vi "lab2_4.vi"() -> ()   [LabVIEW 2017]
panel:
  out "Under Limit":bool
  in  "Slide 2":dbl(slide) scale=78.0..88.0
  out "Over Limit":bool
  in  "Slide":dbl(slide) scale=78.0..88.0
  out "Waveform Chart":T1(graph)
  in  "stop":bool
  out "Numeric":i32
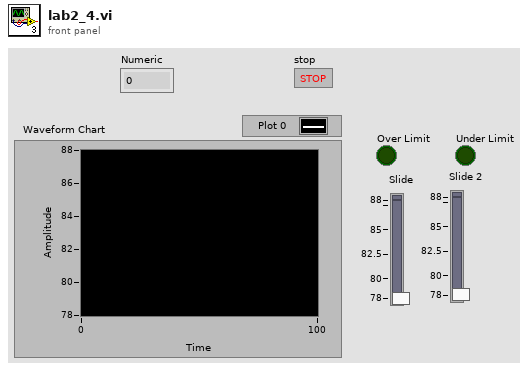
[diagram p1: front panel]
types:
  T1 = cluster{"temperature":dbl, "Slide":dbl, "Slide 2":dbl}
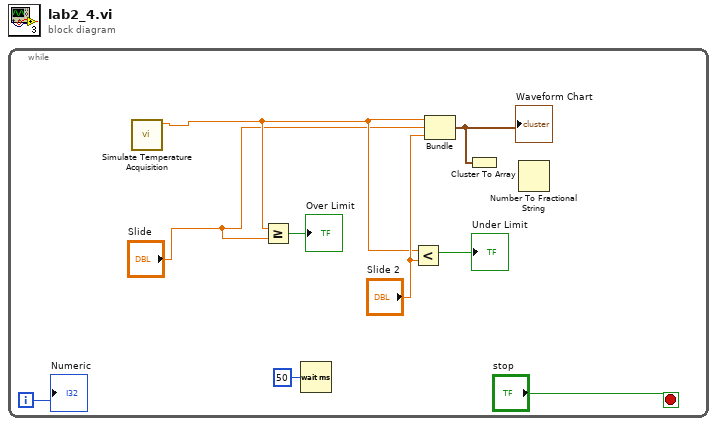
[diagram p0: block diagram]
diagram:
  n1 = while {
    i -> [w9]
    stop <- "stop" stop-if-true
    n2 = call "Simulate Temperature Acquisition.vi"() -> ("temperature"=w3:dbl)  [unwired: 11 in]
    n3 = Greater Or Equal?(x=w3, y="Slide") -> (x >= y?=→"Over Limit":bool)
    n4 = Wait (ms)(milliseconds to wait=u32 50) -> ()  [unwired: 1 out]
    n5 = Less?(x=w3, y="Slide 2") -> (x < y?=→"Under Limit":bool)
    n6 = Bundle("temperature"=w3, "Slide"="Slide", "Slide 2"="Slide 2") -> (w1:T1)  [unwired: 1 in]
    "Waveform Chart" <- w1
    n7 = Cluster To Array(cluster=w1) -> ()  [unwired: 1 out]
    n8 = Number To Fractional String() -> ()  [unwired: 4 in, 1 out]
    "Numeric" <- w9
  }
